vi "2601B线程.vi"() -> (0 "错误输出":errorcluster, 3 "2601B":T1)   [LabVIEW 2021]
uses:
  QueueLib/QueueLib.lvlib
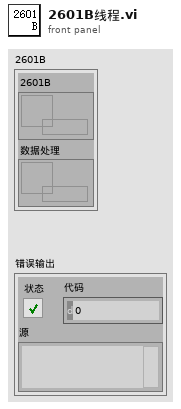
[diagram p1: front panel]
types:
  T1 = cluster{"2601B":refnum<queue>, "数据处理":refnum<queue>}
  T2 = cluster{"队列组[0]":refnum<queue>, "队列组[1]":refnum<queue>}
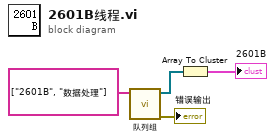
[diagram p0: block diagram]
diagram:
  n1 = call "队列组.vi"("队列名称"=string[] ["2601B", "数据处理"]) -> ("错误输出"=→"错误输出":errorcluster, "队列组"=w2:refnum<queue>[])  [unwired: 9 in]
  n2 = Array To Cluster(array=w2) -> (cluster=→"2601B":T2)
